vi "AssignColors.vi"(6 "Add Spaces?":bool, 9 "Parent":refnum<vi>, 11 "Code":refnum<vi>) -> (2 "Value":string)   [LabVIEW 2016]
uses:
  <vilib>/Utility/miscctls.llb/LVSelectionTypeDef.ctl
  <userlib>/MicroPython/VIs/ColorText/Code.xctl
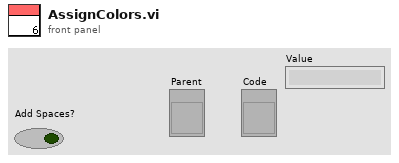
[diagram p1: front panel]
types:
  T1 = typedef "LVSelectionTypeDef.ctl" = cluster{"Selection Start":u32, "Selection End":u32}
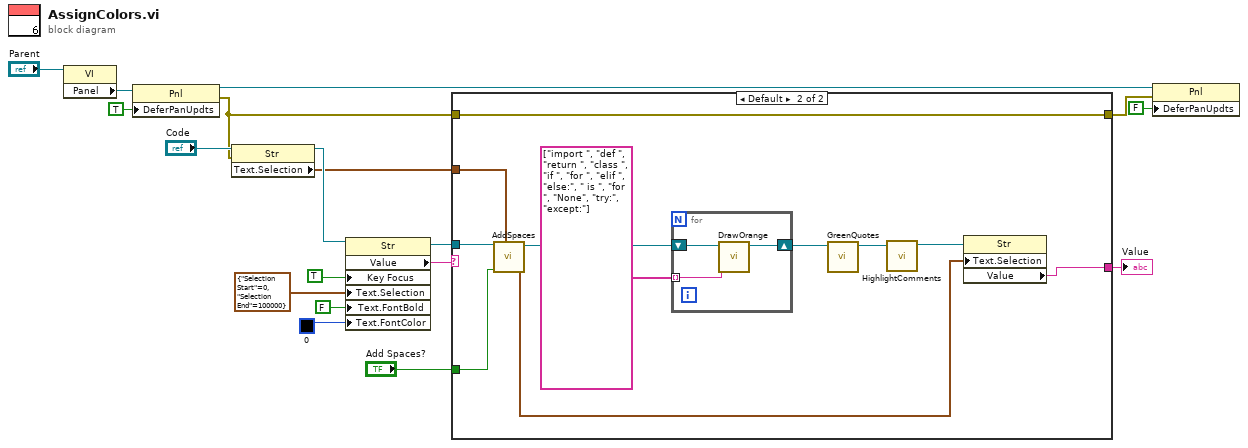
[diagram p0: block diagram]
diagram:
  n1 = property class="VI"(reference="Parent") -> ("Panel"=w10:refnum<vi>)  [unwired: 1 in, 2 out]
  n2 = property class="Pnl"(reference=w10, "DeferPanUpdts"=TRUE ("Defer Panel Updates")) -> (reference out=w7:refnum<vi>, error out=w4:errorcluster)  [unwired: 1 in]
  n3 = property on="Property Node" class="Str"(reference="Code", error in=w4) -> (reference out=w14:refnum<vi>, "Text.Selection"=w13:T1)  [unwired: 1 out]
  n4 = property on="Property Node" class="Str"(reference=w14, "Key Focus"=TRUE, "Text.Selection"=T1 {"Selection Start"=0, "Selection End"=100000}, "Text.FontBold"=FALSE ("Text.Font:Bold"), "Text.FontColor"=u32 0) -> (reference out=w2:refnum<vi>, "Value"=w1:string)  [unwired: 1 in, 1 out]
  n5 = case shown="Default" w1 {
    selector: w1 -> [w20 _]
    tunnel: w2 -> [_ w22]
    tunnel: w13 -> [_ w29]
    tunnel: [w20 w27] -> w11
    tunnel: [w19 w26] -> w5
    tunnel: w4 -> [w19 w26]
    tunnel: "Add Spaces?" -> [_ w23]
    frame "" {
    }
    frame Default {
      n6 = call <userlib>:"AddSpaces.vi"("Text.Selection"=w29, "Add Spaces?"=w23, "String in"=w22) -> ("Cursor"=w25:cluster{u32, u32}, "String out"=w21:refnum<vi>)  [unwired: 7 in]
      n7 = for {
        shift-right: [w33] -> w30
        shift-left: w21 -> [w34]
        tunnel: string[] ["import ", "def ", "return ", "class ", "if ", "for ", "elif ", "else:", " is ", "for ", "None", "try:", "except:"] -> [w32] mode=indexing
        n8 = call <userlib>:"DrawOrange.vi"("Expression"=w32, "String in"=w34) -> ("String out"=w33:refnum<vi>)  [unwired: 9 in]
      }
      n9 = call <userlib>:"GreenQuotes.vi"("String in"=w30) -> ("String out"=w28:refnum<vi>)  [unwired: 10 in]
      n10 = call <userlib>:"HighlightComments.vi"("String in"=w28) -> ("String out"=w24:refnum<vi>)  [unwired: 10 in]
      n11 = property on="Property Node" class="Str"(reference=w24, "Text.Selection"=w25) -> ("Value"=w27:string)  [unwired: 1 in, 2 out]
    }
  }
  "Value" <- w11
  n12 = property class="Pnl"(reference=w7, error in=w5, "DeferPanUpdts"=FALSE ("Defer Panel Updates")) -> ()  [unwired: 2 out]
